vi "PopulateTreeControl.vi"(0 "TreeControl":refnum<vi>, 1 "ObjectAttributes":string[][](array[string]), 2 "ClassAttributes":string[][](array[string]), 3 "ObjectClasses":string[](array[string]), 4 "ClassClasses":string[](array[string]), 5 "error in (no error)":errorcluster) -> (19 "error out":errorcluster)   [LabVIEW 2014, in "ClassWriterGOOP300.lvclass"]
uses:
  <resource>/Framework/Providers/Open_GDS/ClassProviders/Provider_EndevoGOOP300/ClassWriterGOOP300_class/ClassWriterGOOP300.lvclass
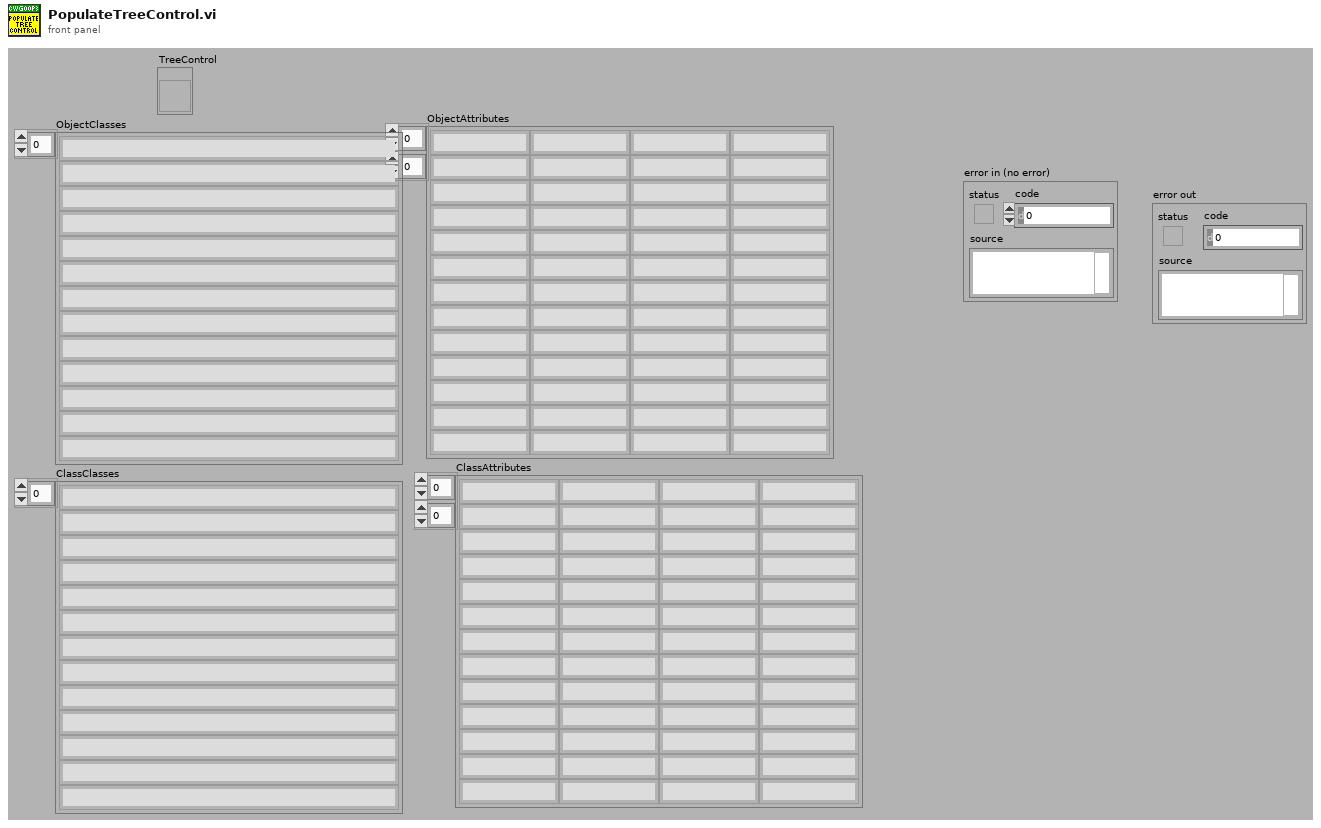
[diagram p1: front panel]
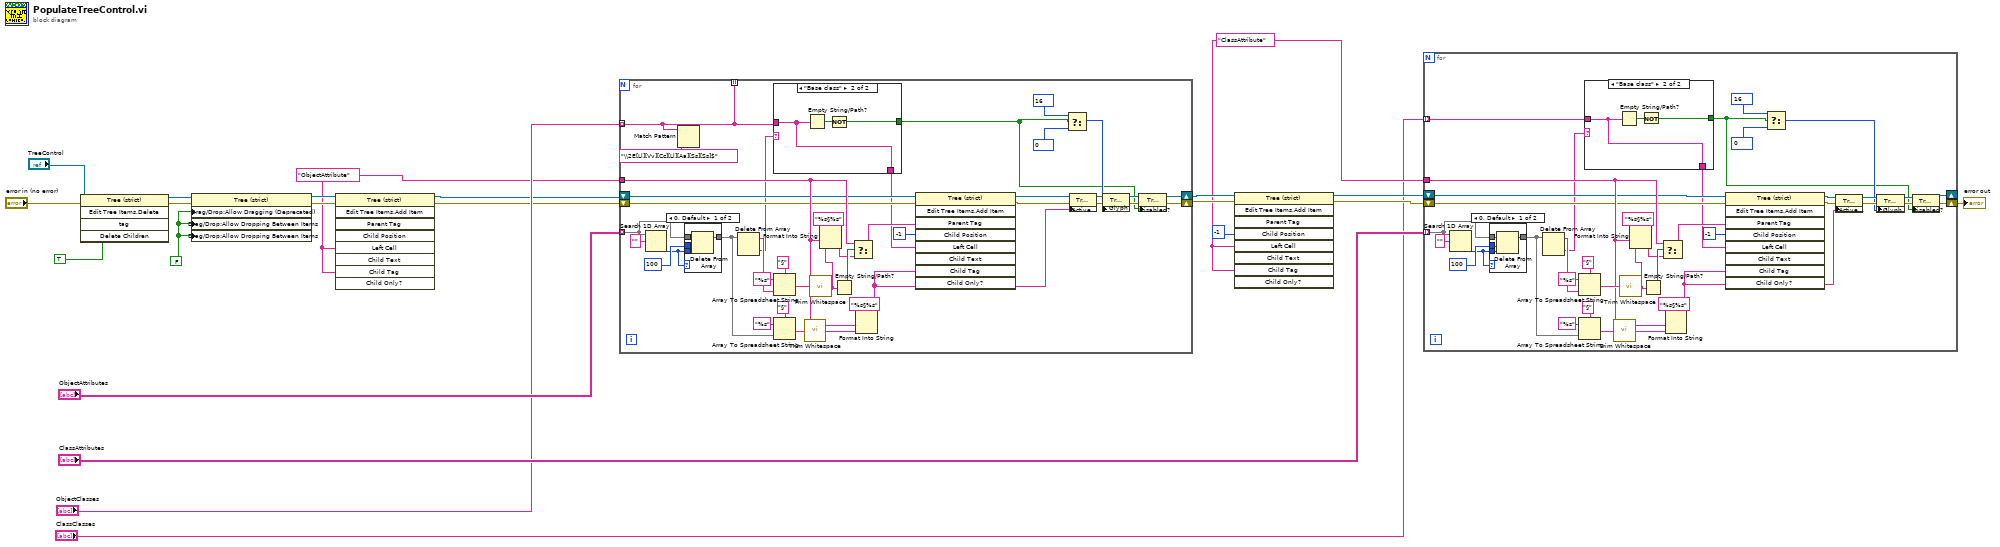
[diagram p0: block diagram]
diagram:
  w4 = "ClassAttribute" ("Left Cell String(Main name)")
  w16 = FALSE ("Drag/Drop:Allow Dragging (Deprecated)")
  w7 = "ObjectAttribute" ("Left Cell String(Main name)")
  n1 = invoke on="Invoke Node" class="Tree (strict)" method="Edit Tree Items.Delete"(reference="TreeControl", error in="error in (no error)", "Delete Children"=TRUE) -> (reference out=w20:refnum<vi>, error out=w19:errorcluster)  [unwired: 2 in, 3 out]
  n2 = property class="Tree (strict)"(reference=w20, error in=w19, "Drag/Drop:Allow Dragging (Deprecated)"=w16, "Drag/Drop:Allow Dropping Between Items"=w16, "Drag/Drop:Allow Dropping Between Items"=w16) -> (reference out=w18:refnum<vi>, error out=w17:errorcluster)
  n3 = invoke on="Invoke Node" class="Tree (strict)" method="Edit Tree Items.Add Item"(reference=w18, error in=w17, "Left Cell"=w7, "Child Tag"=w7) -> (reference out=w6:refnum<vi>, error out=w5:errorcluster)  [unwired: 5 in, 7 out]
  n4 = for {
    shift-right: [w25] -> w14
    shift-left: w5 -> [w42]
    shift-right: [w24] -> w15
    shift-left: w6 -> [w41]
    tunnel: "ObjectAttributes" -> [w61] mode=indexing
    tunnel: w7 -> [w44]
    tunnel: "ObjectClasses" -> [w31] mode=indexing
    tunnel: [w31] -> _ mode=indexing
    n5 = Search 1D Array(1D array=w61, element="") -> (index of element=w50:i32)  [unwired: 1 in]
    n6 = Match Pattern(string=w31, regular expression="\\2E[Ll][Vv][Cc][Ll][Aa][Ss][Ss]$") -> ()  [unwired: 1 in, 4 out]
    n7 = case shown="0, Default" w50 {
      tunnel: w50 -> [w70 _]
      tunnel: w61 -> [w69 w71]
      tunnel: 100 ("length") -> [w68 _]
      tunnel: [w67 w71] -> w51
      frame 0, Default {
        n8 = Delete From Array(array=w69, length=w68, index=w70) -> (array with subset deleted=w67:string[])  [unwired: 1 out]
      }
      frame -1 {
      }
    }
    n9 = Delete From Array(array=w51) -> (deleted portion=w39:string, array with subset deleted=w59:string[])  [unwired: 2 in]
    n10 = case shown="\"Base class\"" w39 {
      selector: w39 -> [w63 _]
      tunnel: [w63 w64] -> w38
      tunnel: w31 -> [_ w64]
      tunnel: [_ w65] -> w23
      frame Default {
      }
      frame "Base class" {
        n11 = Empty String/Path?(string/path=w64) -> (empty?=w66:bool)
        n12 = Not(x=w66) -> (.not. x?=w65:bool)
      }
    }
    n13 = Array To Spreadsheet String(delimiter (Tab)="§", array=w59, 3:"%s" ("format string")) -> (spreadsheet string=w56:string)
    n14 = Array To Spreadsheet String(delimiter (Tab)="§", array=w51, 3:"%s" ("format string")) -> (spreadsheet string=w54:string)
    n15 = call <vilib>:"Trim Whitespace.vi"("string"=w54) -> ("trimmed string"=w45:string)  [unwired: 1 in]
    n16 = call <vilib>:"Trim Whitespace.vi"("string"=w56) -> ("trimmed string"=w48:string)  [unwired: 1 in]
    n17 = Format Into String(format string="%s§%s", w44, w48) -> (resulting string=w47:string)  [unwired: 2 in, 1 out]
    n18 = Empty String/Path?(string/path=w48) -> (empty?=w55:bool)
    n19 = Select(t=w44, s=w55, f=w47) -> (s? t:f=w43:string)
    n20 = Format Into String(format string="%s§%s", w44, w45) -> (resulting string=w32:string)  [unwired: 2 in, 1 out]
    n21 = invoke on="Invoke Node" class="Tree (strict)" method="Edit Tree Items.Add Item"(reference=w41, error in=w42, "Parent Tag"=w43, "Child Position"=-1, "Left Cell"=w38, "Child Tag"=w32) -> (reference out=w34:refnum<vi>, error out=w33:errorcluster)  [unwired: 3 in, 7 out]
    n22 = Select(t=16, s=w23, f=0) -> (s? t:f=w28:i32)
    n23 = property class="Tree (strict)"(reference=w34, error in=w33, "Active Item Tag"=w32) -> (reference out=w36:refnum<vi>, error out=w35:errorcluster)
    n24 = property class="Tree (strict)"(reference=w36, error in=w35, "Glyph"=w28) -> (reference out=w27:refnum<vi>, error out=w26:errorcluster)
    n25 = property class="Tree (strict)"(reference=w27, error in=w26, "Disabled?"=w23) -> (reference out=w24:refnum<vi>, error out=w25:errorcluster)
  }
  n26 = invoke on="Invoke Node" class="Tree (strict)" method="Edit Tree Items.Add Item"(reference=w15, error in=w14, "Child Position"=-1, "Left Cell"=w4, "Child Tag"=w4) -> (reference out=w3:refnum<vi>, error out=w2:errorcluster)  [unwired: 4 in, 7 out]
  n27 = for {
    shift-right: [w74] -> w11
    shift-left: w2 -> [w90]
    shift-right: [w73] -> _
    shift-left: w3 -> [w89]
    tunnel: "ClassAttributes" -> [w109] mode=indexing
    tunnel: w4 -> [w92]
    tunnel: "ClassClasses" -> [w80] mode=indexing
    n28 = Search 1D Array(1D array=w109, element="") -> (index of element=w98:i32)  [unwired: 1 in]
    n29 = case shown="0, Default" w98 {
      tunnel: w98 -> [w118 _]
      tunnel: w109 -> [w117 w119]
      tunnel: 100 ("length") -> [w116 _]
      tunnel: [w115 w119] -> w99
      frame 0, Default {
        n30 = Delete From Array(array=w117, length=w116, index=w118) -> (array with subset deleted=w115:string[])  [unwired: 1 out]
      }
      frame -1 {
      }
    }
    n31 = Delete From Array(array=w99) -> (deleted portion=w87:string, array with subset deleted=w107:string[])  [unwired: 2 in]
    n32 = Array To Spreadsheet String(delimiter (Tab)="§", array=w107, 3:"%s" ("format string")) -> (spreadsheet string=w104:string)
    n33 = Array To Spreadsheet String(delimiter (Tab)="§", array=w99, 3:"%s" ("format string")) -> (spreadsheet string=w102:string)
    n34 = case shown="\"Base class\"" w87 {
      selector: w87 -> [w111 _]
      tunnel: [w111 w112] -> w86
      tunnel: w80 -> [_ w112]
      tunnel: [_ w113] -> w72
      frame Default {
      }
      frame "Base class" {
        n35 = Empty String/Path?(string/path=w112) -> (empty?=w114:bool)
        n36 = Not(x=w114) -> (.not. x?=w113:bool)
      }
    }
    n37 = call <vilib>:"Trim Whitespace.vi"("string"=w102) -> ("trimmed string"=w93:string)  [unwired: 1 in]
    n38 = call <vilib>:"Trim Whitespace.vi"("string"=w104) -> ("trimmed string"=w96:string)  [unwired: 1 in]
    n39 = Format Into String(format string="%s§%s", w92, w96) -> (resulting string=w95:string)  [unwired: 2 in, 1 out]
    n40 = Empty String/Path?(string/path=w96) -> (empty?=w103:bool)
    n41 = Select(t=w92, s=w103, f=w95) -> (s? t:f=w91:string)
    n42 = Format Into String(format string="%s§%s", w92, w93) -> (resulting string=w81:string)  [unwired: 2 in, 1 out]
    n43 = invoke on="Invoke Node" class="Tree (strict)" method="Edit Tree Items.Add Item"(reference=w89, error in=w90, "Parent Tag"=w91, "Child Position"=-1, "Left Cell"=w86, "Child Tag"=w81) -> (reference out=w83:refnum<vi>, error out=w82:errorcluster)  [unwired: 3 in, 7 out]
    n44 = Select(t=16, s=w72, f=0) -> (s? t:f=w78:i32)
    n45 = property class="Tree (strict)"(reference=w83, error in=w82, "Active Item Tag"=w81) -> (reference out=w85:refnum<vi>, error out=w84:errorcluster)
    n46 = property class="Tree (strict)"(reference=w85, error in=w84, "Glyph"=w78) -> (reference out=w76:refnum<vi>, error out=w75:errorcluster)
    n47 = property class="Tree (strict)"(reference=w76, error in=w75, "Disabled?"=w72) -> (reference out=w73:refnum<vi>, error out=w74:errorcluster)
  }
  "error out" <- w11
